vi "Reset.vi"(8 "error in (no error)":errorcluster, 11 "PID in":refnum<class "PID.lvclass">) -> (0 "error out":errorcluster, 3 "PID out":refnum<class "PID.lvclass">)   [LabVIEW 2020, in "IG PID.lvlib" / "PID.lvclass"]
uses:
  PID.lvclass
  PID.lvclass/PID.ctl
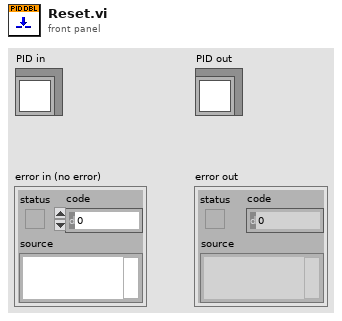
[diagram p1: front panel]
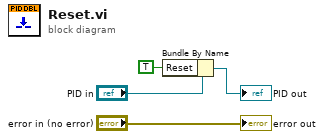
[diagram p0: block diagram]
diagram:
  n1 = Bundle By Name(cluster="PID in", "Reset"=TRUE) -> (→"PID out":refnum<class "PID.lvclass">)
  "error out" <- "error in (no error)"
